vi "Create Reaper.vi"(6 "Additional Applications to Register":string[](array[string])) -> ()   [LabVIEW 2015, in "Reaper.lvclass"]
uses:
  Reaper.lvclass
  Reaper.lvclass/Reaper.ctl
  Reaper Singleton.vi
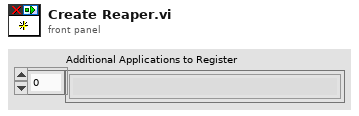
[diagram p1: front panel]
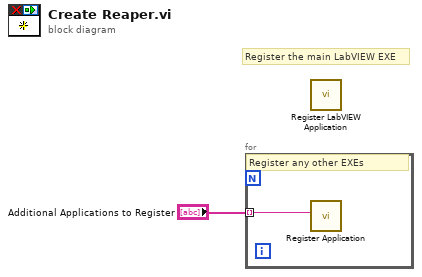
[diagram p0: block diagram]
diagram:
  # "Register the main LabVIEW EXE"
  n1 = for {
    tunnel: "Additional Applications to Register" -> [w2] mode=indexing
    # "Register any other EXEs"
    n2 = call "Register Application.vi"("Application to Register"=w2) -> ()  [unwired: 11 in]
  }
  n3 = call "Register LabVIEW Application.vi"() -> ()  [unwired: 12 in]
